vi "Gyro Steer.vi"(4 "Reinit?":bool, 6 "Steer PID Gains":T1, 8 "Gyro Tolerance":dbl, 9 "X Min Output":dbl, 10 "X Max Output":dbl, 11 "Target Heading":dbl) -> (2 "Finished":bool, 3 "X Out":dbl)   [LabVIEW 2017]
uses:
  Common Code/PID Gains Cluster.ctl
  <vilib>/Rock Robotics/WPI/ThirdParty/Sensors/navX/_TypeDefs/FRIC_navX_DeviceNumbersTypeDef.ctl
  <vilib>/addons/control/pid/pid.llb/PID (DBL).vi
  <vilib>/addons/control/pid/NI_PID_pid.lvlib
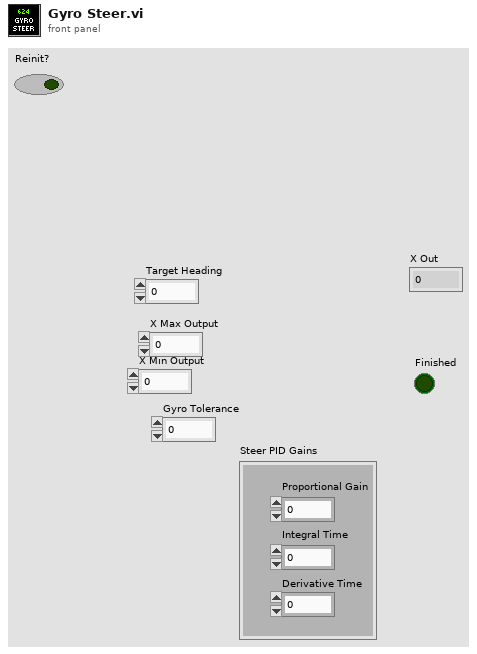
[diagram p1: front panel]
types:
  T1 = typedef "PID Gains Cluster.ctl" = cluster{"Integral Time":dbl, "Proportional Gain":dbl, "Derivative Time":dbl}
  T2 = typedef "FRIC_navX_DeviceNumbersTypeDef.ctl" = enum16{"Dev0", "Dev1", "Dev2", "Dev3"}
  T3 = cluster{"Yaw":dbl, "Roll":dbl, "Pitch":dbl, "Heading":dbl, "Fused Heading":dbl}
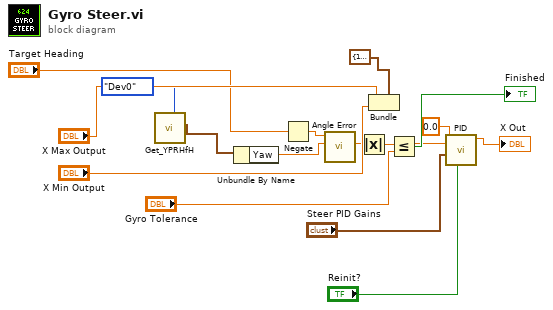
[diagram p0: block diagram]
diagram:
  n1 = call <vilib>:"Get_YPRHfH.vi"("Device Number"=FRIC_navX_DeviceNumbersTypeDef."Dev0") -> ("YRPHfH"=w2:T3)  [unwired: 10 in]
  n2 = Unbundle By Name(w2) -> ("Yaw"=w8:dbl)
  n3 = Negate(x="Target Heading") -> (-x=w10:dbl)
  n4 = call "Angle Error.vi"("Angle"=w8, "Target Angle"=w10) -> ("Error"=w11:dbl)  [unwired: 9 in]
  n5 = Absolute Value(x=w11) -> (abs(x)=w12:dbl)
  n6 = Bundle(cluster=cluster{dbl, dbl} {100.0, -100.0}, "X Max Output", "X Min Output") -> ()  [unwired: 1 out]
  n7 = Less Or Equal?(x=w12, y="Gyro Tolerance") -> (x <= y?=→"Finished":bool)
  n8 = call-poly <vilib>:"PID.vi"("reinitialize? (F)"="Reinit?", "PID gains"="Steer PID Gains", "process variable"=w11, "setpoint"=0.0) -> ("output"=→"X Out":dbl)  [unwired: 6 in, 1 out]
